vi "CFO Correction.vi"(6 "fs":dbl=7680000.0, 8 "CFOest (freq)":dbl[](array[numeric]), 10 "Index":i32, 11 "Input":cdb[](array[numeric])) -> (3 "Output":cdb[](array[numeric]))   [LabVIEW 2022 SP3]
doc: "Corrects Carrier Frequency Offset (CFO)"
uses:
  <vilib>/Analysis/1siggen.llb/Ramp Pattern by Samples.vi
  <vilib>/Analysis/NI_AALBase.lvlib
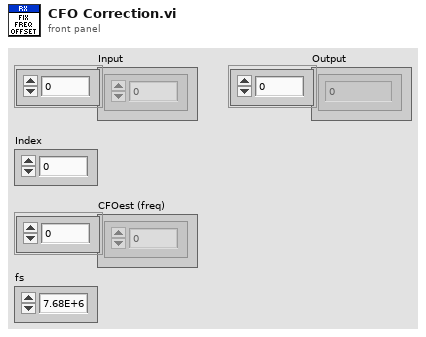
[diagram p1: front panel]
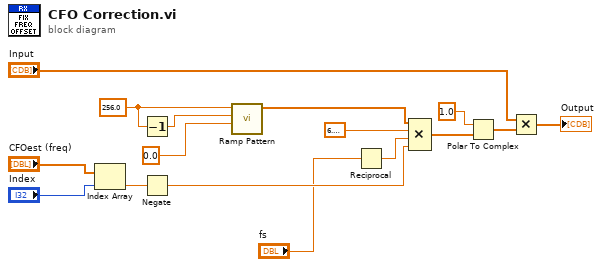
[diagram p0: block diagram]
diagram:
  w9 = 256.0 ("start")
  n1 = Index Array(array="CFOest (freq)", index="Index") -> (element=w12:dbl)
  n2 = Decrement(x=w9) -> (x-1=w6:dbl)
  n3 = Negate(x=w12) -> (-x=w13:dbl)
  n4 = call-poly <vilib>:"Ramp Pattern.vi"("start"=0.0, "end"=w6, "samples"=w9) -> ("Ramp Pattern"=w4:dbl[])  [unwired: 7 in, 1 out]
  n5 = Reciprocal(x="fs") -> (1/x=w8:dbl)
  n6 = Compound Arithmetic op=MULTIPLY(w4, 6.283185307179586, w8, w13) -> (w3:dbl[])
  n7 = Polar To Complex(1:w3, 2:1.0 ("value")) -> (0:w15:cdb[])
  n8 = Multiply(x="Input", y=w15) -> (x*y=→"Output":cdb[])
